vi "SetupWrapper.vi"(10 "Actor":T1, 11 "Layer":T6) -> (2 "Actor":T1, 3 "Layer":T6, 4 "Error":errorcluster)   [LabVIEW 2020, in "jettl.lvlib"]
uses:
  jettl.lvlib
  Actor/Actor.lvclass
  Layer.ctl
  Msg/Msg.lvclass
  Origin.ctl
  Metadata/Metadata.lvclass
  Lifecycle.ctl
  MsgAttribs.ctl
  Msg.ctl
  PostSetup.ctl
  PreSetup.ctl
  MsgNames.ctl
  ActorAttribs.ctl
  ChildActors.ctl
  Actor.ctl
  MsgExecuteType.ctl
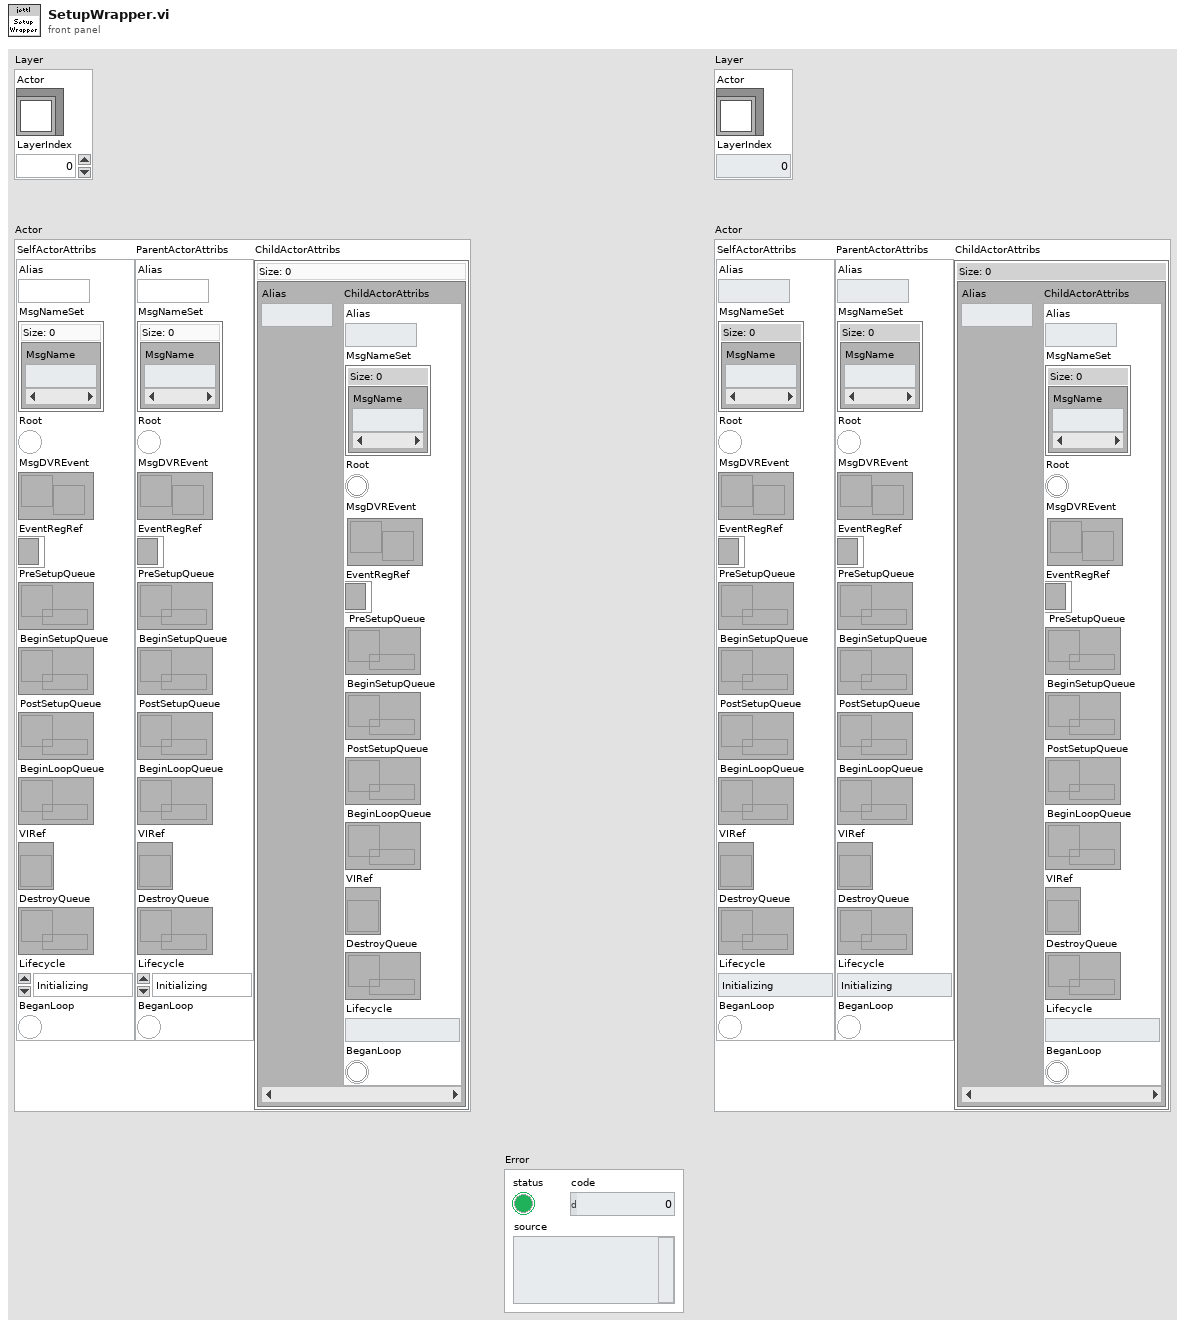
[diagram p1: front panel]
types:
  T1 = typedef "jettl.lvlib/Actor.ctl" = cluster{"SelfActorAttribs":T2, "ParentActorAttribs":T2, "ChildActorAttribs":T5}
  T2 = typedef "jettl.lvlib/ActorAttribs.ctl" = cluster{"Alias":string, "MsgNameSet":T3, "Root":bool, "MsgDVREvent":refnum<user-event>, "EventRegRef":refnum<event-registration>, "PreSetupQueue":refnum<queue>, "BeginSetupQueue":refnum<queue>, "PostSetupQueue":refnum<queue>, "BeginLoopQueue":refnum<queue>, "VIRef":refnum<vi>, "DestroyQueue":refnum<queue>, "Lifecycle":T4, "BeganLoop":bool}
  T3 = typedef "jettl.lvlib/MsgNames.ctl" = set{string}
  T4 = typedef "jettl.lvlib/Lifecycle.ctl" = enum16{"Initializing", "SettingUp", "Starting", "Running", "Stopping", "TearingDown", "Terminated"}
  T5 = typedef "jettl.lvlib/ChildActors.ctl" = map{string, T2}
  T6 = typedef "jettl.lvlib/Layer.ctl" = cluster{"Actor":refnum<class "Actor.lvclass">, "LayerIndex":u8}
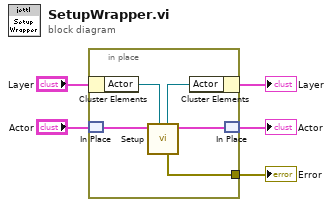
[diagram p0: block diagram]
diagram:
  n1 = in-place {
    in-place-border: [w8] -> w5
    n2 = in-place-cluster #1("Layer") -> ("Actor"=w10:refnum<class "Actor.lvclass">)
    n3 = in-place-match #2("Actor") -> (w7:T1)
    n4 = call-dynamic "Setup.vi"(7:"Actor"=w10, 11:"Actor"=w7) -> (3:"Actor"=w6:T1, "Error"=w8:errorcluster, 5:"Actor"=w9:refnum<class "Actor.lvclass">)  [unwired: 7 in]
    n5 = in-place-cluster #1("Actor"=w9) -> (→"Layer":T6)
    n6 = in-place-match #2(w6) -> (→"Actor":T1)
  }
  "Error" <- w5
